vi "Read FSM Queue.vi"(8 "error in (no error)":errorcluster, 11 "FSM Data in":T1={"FSM State"=enum."App_Close", "Spectrum Reader"="Reader", "Recording"=FALSE, "IP Address"="", "Raw Data Reader"=""}) -> (0 "error out":errorcluster, 2 "FSM State":T2=enum."App_Idle", 3 "FSM Data out":T1={"FSM State"=enum."App_Close", "Spectrum Reader"="Reader", "Recording"=FALSE, "IP Address"="", "Raw Data Reader"=""})   [LabVIEW 2017]
uses:
  FSM Data.ctl
  FSM States.ctl
  Application Globals.vi
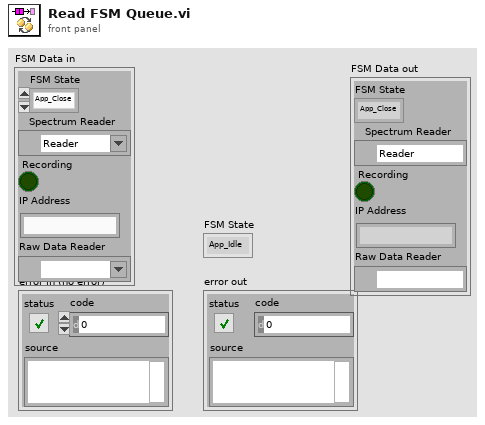
[diagram p1: front panel]
types:
  T1 = typedef "FSM Data.ctl" = cluster{"FSM State":T2, "Spectrum Reader":refnum<k21>, "Recording":bool, "IP Address":string, "Raw Data Reader":refnum<k21>}
  T2 = typedef "FSM States.ctl" = enum16{"App_Disconnect", "App_Idle", "App_Connect", "App_Close", "APP_Init", "App_Logging", "App_SetRecordStateOn", "App_SetRecordStateOff"}
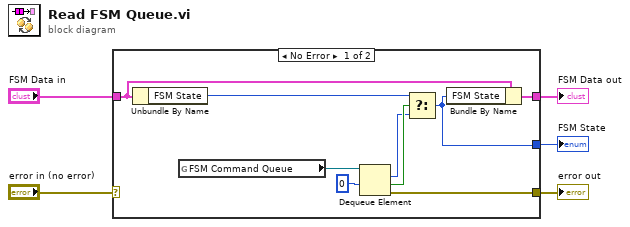
[diagram p0: block diagram]
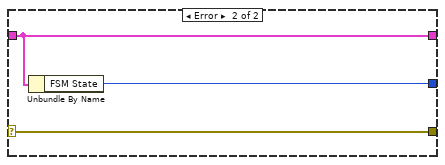
[diagram p2: hidden frame]
diagram:
  n1 = case shown="No Error" "error in (no error)" {
    selector: "error in (no error)" -> [_ w17]
    tunnel: "FSM Data in" -> [w9 w15]
    tunnel: [w8 w16] -> w2
    tunnel: [w7 w15] -> w3
    tunnel: [w6 w17] -> w4
    frame No Error {
      n2 = Unbundle By Name(w9) -> ("FSM State"=w10:T2)
      n3 = global read "Application Globals.vi" "FSM Command Queue"() -> (w14:refnum<queue>)
      n4 = Dequeue Element(queue=w14, timeout in ms (-1)=0) -> (element=w11:T2, timed out?=w12:bool, error out=w6:errorcluster)  [unwired: 1 in, 1 out]
      n5 = Select(t=w10, s=w12, f=w11) -> (s? t:f=w8:T2)
      n6 = Bundle By Name(cluster=w9, "FSM State"=w8) -> (w7:T1)
    }
    frame Error {
      n7 = Unbundle By Name(w15) -> ("FSM State"=w16:T2)
    }
  }
  "error out" <- w4
  "FSM Data out" <- w3
  "FSM State" <- w2
